vi "element_data_write.vi"(7 "container_name":string, 8 "error in (no error)":errorcluster, 10 "Variant":variant, 11 "Refnum in":T1) -> (0 "error out":errorcluster, 3 "Refnum out":T1)   [LabVIEW 2015, in "ini_work_Library.lvlib"]
uses:
  ini_work_Library.lvlib
  <vilib>/Utility/config.llb/Config Data RefNum.ctl
  <vilib>/Utility/config.llb/Write Key (I32).vi
  <vilib>/Utility/config.llb/Write Key (Double).vi
  <vilib>/Utility/config.llb/Write Key (Boolean).vi
  <vilib>/Utility/config.llb/Write Key (String).vi
  <vilib>/Utility/config.llb/Write Key (Path).vi
  <vilib>/Utility/config.llb/NI_LVConfig.lvlib
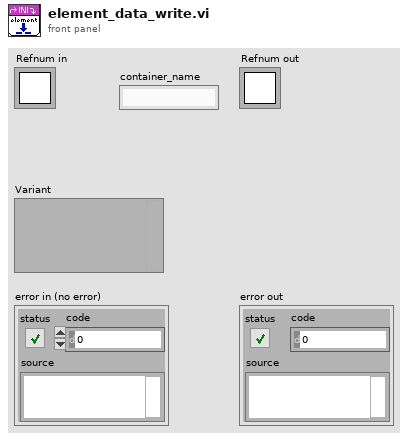
[diagram p1: front panel]
types:
  T1 = typedef "NI_LVConfig.lvlib/Config Data RefNum.ctl" = refnum<k1>
  T2 = typedef "Type Descriptor Enumeration__ogtk.ctl" = enum8{"<Null>", "I8", "I16", "I32", "I64", "U8", "U16", "U32", "U64", "SGL", "DBL", "EXT", "CSG", "CDB", "CXT", "0x0F", "0x10", "0x11", "0x12", "0x13", "0x14", "Enum U8", "Enum U16", "Enum U32", "Enum U64", "SGL PQ", "DBL PQ", "EXT PQ", "CSG PQ", "CDB PQ", "CXT PQ", "0x1F", "0x20", "Boolean", "0x22", "0x23", "0x24", "0x25", "0x26", "0x27", "0x28", "0x29", "0x2A", "0x2B", "0x2C", "0x2D", "0x2E", "0x2F", "String", "0x31", "Path", "Pict", "0x34", "0x35", "0x36", "DAQ", "0x38", "0x39", "0x3A", "0x3B", "0x3C", "0x3D", "0x3E", "0x3F", "Array", "0x41", "0x42", "0x43", "0x44", "0x45", "0x46", "0x47", "0x48", "0x49", "0x4A", "0x4B", "0x4C", "0x4D", "0x4E", "0x4F", "Cluster", "0x51", "0x52", "Variant", "Waveform", "0x55", "0x56", "0x57", "0x58", "0x59", "0x5A", "0x5B", "0x5C", "0x5D", "0x5E", "Fixed Point", "0x60", "0x61", "0x62", "0x63", "0x64", "0x65", "0x66", "0x67", "0x68", "0x69", "0x6A", "0x6B", "0x6C", "0x6D", "0x6E", "0x6F", "Refnum", "0x71", "0x72", "Set Collection", "Map Collection"}
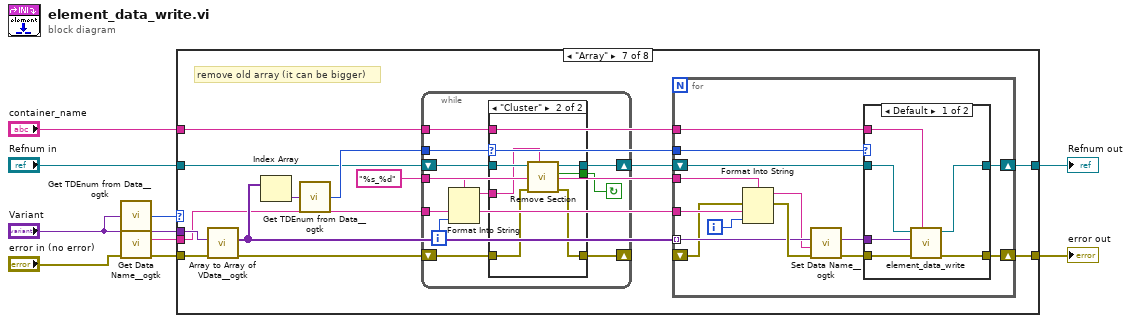
[diagram p0: block diagram]
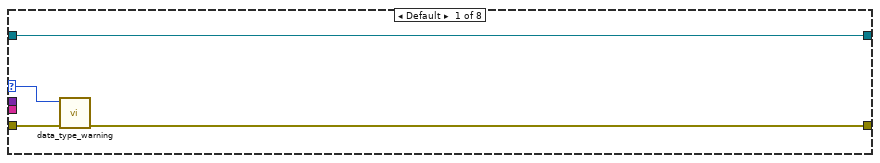
[diagram p2: hidden frame]
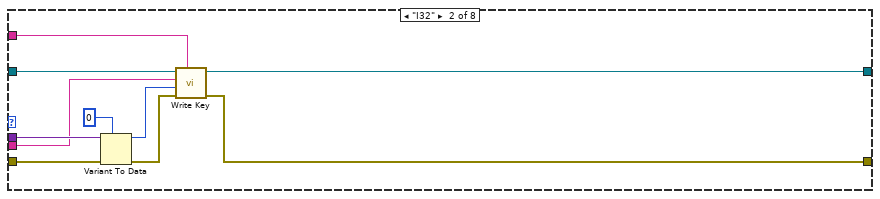
[diagram p3: hidden frame]
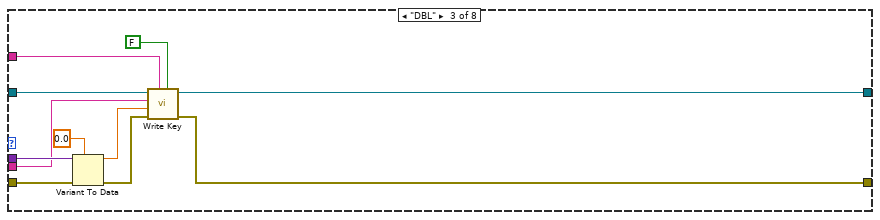
[diagram p4: hidden frame]
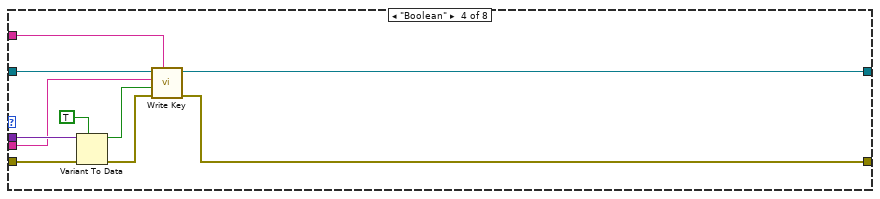
[diagram p5: hidden frame]
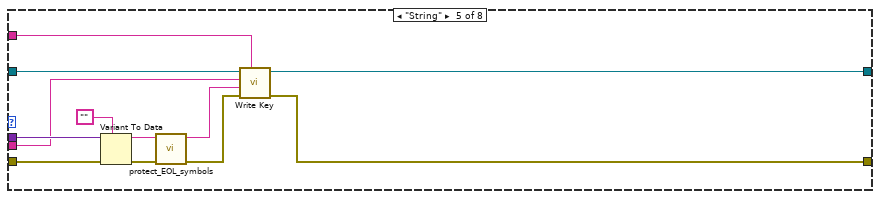
[diagram p6: hidden frame]
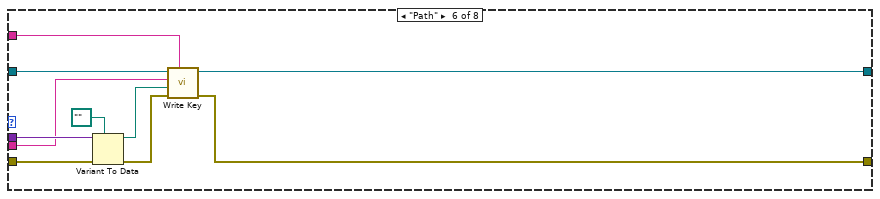
[diagram p7: hidden frame]
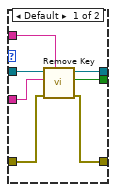
[diagram p8: hidden frame]
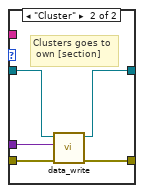
[diagram p9: hidden frame]
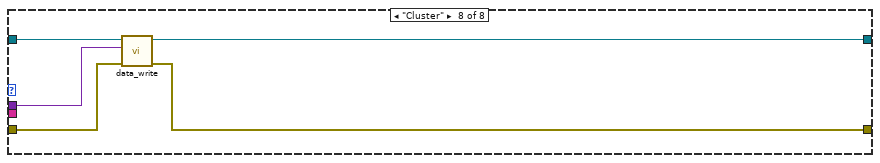
[diagram p10: hidden frame]
diagram:
  n1 = call <userlib>:"Get TDEnum from Data__ogtk.vi"("Data"="Variant") -> ("Type Descriptor Enumeration"=w1:T2)  [unwired: 4 in]
  n2 = call <userlib>:"Get Data Name__ogtk.vi"("error in (no error)"="error in (no error)", "Data"="Variant") -> ("error out"=w7:errorcluster, "Data Name"=w6:string, "Data dup"=w5:variant)  [unwired: 7 in]
  n3 = case shown="\"Array\"" w1 {
    selector: w1 -> [w13 _ _ _ _ _ _ _]
    tunnel: "Refnum in" -> [w14 w21 w32 w42 w54 w64 w71 w133]
    tunnel: w5 -> [_ w24 w35 w45 w57 w67 w78 w132]
    tunnel: w6 -> [_ w19 w30 w40 w52 w62 w69 _]
    tunnel: w7 -> [w12 w23 w34 w44 w56 w66 w77 w131]
    tunnel: "container_name" -> [_ w20 w31 w41 w53 w63 w72 _]
    tunnel: [w14 w16 w27 w37 w51 w60 w80 w130] -> w9
    tunnel: [w11 w15 w26 w36 w50 w59 w79 w129] -> w10
    frame Default {
      n4 = call "data_type_warning.vi"("error in (no error)"=w12, "Type Descriptor Enumeration"=w13) -> ("error out"=w11:errorcluster)  [unwired: 9 in]
    }
    frame "I32" {
      n5 = Variant To Data(error in=w23, type=0, Variant=w24) -> (data=w18:i32, error out=w17:errorcluster)
      n6 = call-poly <vilib>:"Write Key.vi"("section"=w20, "error in (no error)"=w17, "value"=w18, "key"=w19, "refnum"=w21) -> ("error out"=w15:errorcluster, "refnum out"=w16:T1)  [unwired: 4 in, 1 out]
    }
    frame "DBL" {
      n7 = Variant To Data(error in=w34, type=0.0, Variant=w35) -> (data=w29:dbl, error out=w28:errorcluster)
      n8 = call-poly <vilib>:"Write Key.vi"("use system decimal point (T)"=FALSE, "section"=w31, "error in (no error)"=w28, "value"=w29, "key"=w30, "refnum"=w32) -> ("error out"=w26:errorcluster, "refnum out"=w27:T1)  [unwired: 3 in, 1 out]
    }
    frame "Boolean" {
      n9 = Variant To Data(error in=w44, type=TRUE, Variant=w45) -> (data=w39:bool, error out=w38:errorcluster)
      n10 = call-poly <vilib>:"Write Key.vi"("section"=w41, "error in (no error)"=w38, "value"=w39, "key"=w40, "refnum"=w42) -> ("error out"=w36:errorcluster, "refnum out"=w37:T1)  [unwired: 4 in, 1 out]
    }
    frame "String" {
      n11 = Variant To Data(error in=w56, type="", Variant=w57) -> (data=w49:string, error out=w47:errorcluster)
      n12 = call "protect_EOL_symbols.vi"("error in (no error)"=w47, "String"=w49) -> ("error out"=w46:errorcluster, "result string"=w48:string)  [unwired: 8 in]
      n13 = call-poly <vilib>:"Write Key.vi"("section"=w53, "error in (no error)"=w46, "value"=w48, "key"=w52, "refnum"=w54) -> ("error out"=w50:errorcluster, "refnum out"=w51:T1)  [unwired: 4 in, 1 out]
    }
    frame "Path" {
      n14 = Variant To Data(error in=w66, type=path "", Variant=w67) -> (data=w58:path, error out=w61:errorcluster)
      n15 = call-poly <vilib>:"Write Key.vi"("section"=w63, "error in (no error)"=w61, "value"=w58, "key"=w62, "refnum"=w64) -> ("error out"=w59:errorcluster, "refnum out"=w60:T1)  [unwired: 4 in, 1 out]
    }
    frame "Array" {
      w68 = "%s_%d"
      # "remove old array (it can be bigger)"
      n16 = call <userlib>:"Array to Array of VData__ogtk.vi"("error in (no error)"=w77, "MultiD Array"=w78) -> ("error out"=w73:errorcluster, "1D Array of Variants"=w76:variant[])  [unwired: 8 in]
      n17 = Index Array(array=w76) -> (element=w75:variant)  [unwired: 1 in]
      n18 = call <userlib>:"Get TDEnum from Data__ogtk.vi"("Data"=w75) -> ("Type Descriptor Enumeration"=w74:T2)  [unwired: 4 in]
      n19 = while {
        tunnel: w74 -> [w91]
        tunnel: w68 -> [w90]
        shift-right: [w87] -> w70
        shift-left: w71 -> [w88]
        shift-right: [w85] -> _
        shift-left: w73 -> [w86]
        tunnel: w72 -> [w82]
        tunnel: w69 -> [w81]
        i -> [w89]
        stop <- w83 continue-if-true
        n20 = Format Into String(format string=w90, w81, w89) -> (resulting string=w84:string)  [unwired: 2 in, 1 out]
        n21 = case shown="\"Cluster\"" w91 {
          tunnel: w88 -> [w98 w104]
          tunnel: [w93 w103] -> w87
          tunnel: [w92 w102] -> w83
          tunnel: w86 -> [w95 w101]
          tunnel: [w94 w100] -> w85
          tunnel: w82 -> [w97 _]
          tunnel: w84 -> [w96 w99]
          frame Default {
            n22 = call <vilib>:"Remove Key.vi"("section"=w97, "error in (no error)"=w95, "key"=w96, "refnum"=w98) -> ("error out"=w94:errorcluster, "found?"=w92:bool, "refnum out"=w93:T1)  [unwired: 5 in]
          }
          frame "Cluster" {
            n23 = call <vilib>:"Remove Section.vi"("section"=w99, "error in (no error)"=w101, "refnum"=w104) -> ("error out"=w100:errorcluster, "section exists?"=w102:bool, "refnum out"=w103:T1)  [unwired: 6 in]
          }
        }
      }
      n24 = for {
        shift-right: [w115] -> w80
        shift-left: w70 -> [w109]
        shift-right: [w116] -> w79
        shift-left: _ -> [w108]
        tunnel: w76 -> [w113] mode=indexing
        tunnel: w69 -> [w110]
        tunnel: w72 -> [w107]
        tunnel: w74 -> [w106]
        tunnel: w68 -> [w105]
        i -> [w117]
        n25 = Format Into String(format string=w105, error in=w108, w110, w117) -> (resulting string=w112:string, error out=w114:errorcluster)  [unwired: 1 in]
        n26 = call <userlib>:"Set Data Name__ogtk.vi"("error in (no error)"=w114, "Data Name"=w112, "Data"=w113) -> ("Renamed Data"=w111:variant)  [unwired: 7 in, 1 out]
        n27 = case shown="Default" w106 {
          tunnel: w114 -> [w123 w128]
          tunnel: [w122 w127] -> w116
          tunnel: w109 -> [w119 w125]
          tunnel: [w118 w124] -> w115
          tunnel: w111 -> [w121 w126]
          tunnel: w107 -> [w120 _]
          frame Default {
            n28 = call "element_data_write.vi"("container_name"=w120, "error in (no error)"=w123, "Variant"=w121, "Refnum in"=w119) -> ("error out"=w122:errorcluster, "Refnum out"=w118:T1)  [unwired: 6 in]
          }
          frame "Cluster" {
            # "Clusters goes to\n own [section]"
            n29 = call "data_write.vi"("error in (no error)"=w128, "data"=w126, "ini_file_refnum"=w125) -> ("error out"=w127:errorcluster, "ini_file_refnum_out"=w124:T1)  [unwired: 7 in]
          }
        }
      }
    }
    frame "Cluster" {
      n30 = call "data_write.vi"("error in (no error)"=w131, "data"=w132, "ini_file_refnum"=w133) -> ("error out"=w129:errorcluster, "ini_file_refnum_out"=w130:T1)  [unwired: 7 in]
    }
  }
  "error out" <- w10
  "Refnum out" <- w9
